vi "点位与索引匹配.vi"(9 "匹配索引号":i32, 10 "配置信息":string[][](table)=[["名称", "点位", "索引号", "逻辑取反"], ["启动按钮", "X100", "0", "0"], ["复位按钮", "X101", "1", "0"], ["暂停按钮", "X102", "2", "0"], ["操作侧安全光栅", "X103", "3", "0"], ["后侧安全光栅", "X104", "4", "0"], ["上层真空检知", "X105", "5", "0"], ["下层真空检知", "X106", "6", "0"], ["上层感应sensor", "X107", "7", "0"], ["下层感应sensor", "X110", "8", "0"], ["传送抓手气缸前位", "X111", "9", "0"], ["传送抓手气缸后位", "X112", "10", "0"], ["上层产品定位气缸前位", "X113", "11", "0"], ["上层产品定位气缸后位", "X114", "12", "0"], ["下层产品定位气缸前位", "X115", "13", "0"], ["下层产品定位气缸后位", "X116", "14", "0"], ["抓手感应产品sensor", "X117", "15", "0"], ["起子1真空检知", "X120", "16", "0"], ["起子2真空检知", "X121", "17", "0"], ["起子3真空检知", "X122", "18", "0"], ["起子4真空检知", "X123", "19", "0"], ["feed01感应sensor", "X124", "20", "0"], ["feed02感应sensor", "X125", "21", "0"], ["feed03感应sensor", "X126", "22", "0"], ["feed04感应sensor", "X127", "23", "0"], ["动子1和2统一坐标sensor", "X130", "24", "0"], ["动子3和4统一坐标sensor", "X131", "25", "0"], ["前后侧统一坐标sensor", "X132", "26", "0"], ["上站允许取料信号", "X133", "27", "0"], ["下站允许投料信号", "X134", "28", "0"], ["上站请求信号", "X135", "29", "0"], ["下站答复信号", "X136", "30", "0"]]) -> (2 "ERROR 2":string)   [LabVIEW 2012]
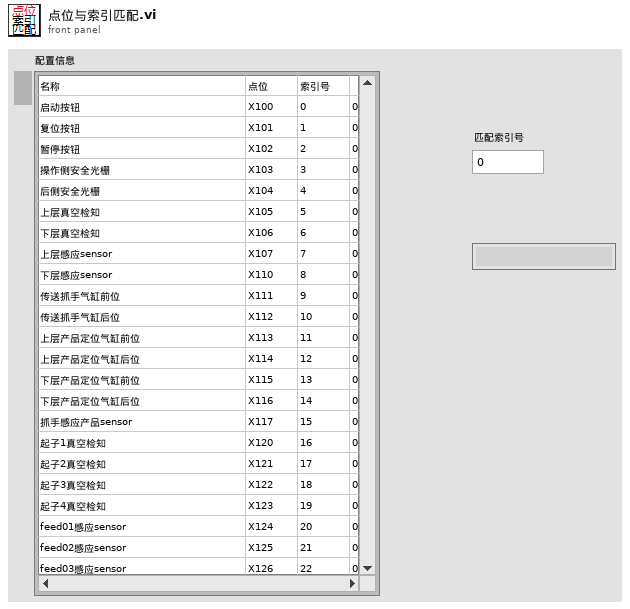
[diagram p1: front panel]
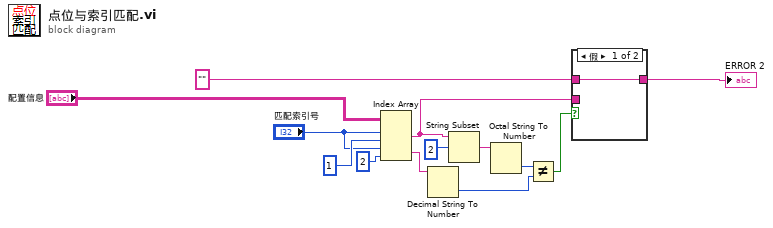
[diagram p0: block diagram]
diagram:
  n1 = Index Array(array="配置信息", index (row) #1="匹配索引号", index (col) #1=1 ("禁用的索引 (列)"), index (row) #2="匹配索引号", index (col) #2=2 ("索引 (列)")) -> (element #1=w1:string, element #2=w4:string)
  n2 = Decimal String To Number(string=w4) -> (number=w7:i32)  [unwired: 2 in, 1 out]
  n3 = String Subset(string=w1, offset (0)=2 ("长度（剩余）")) -> (substring=w9:string)  [unwired: 1 in]
  n4 = Octal String To Number(4:w9) -> (0:w8:u32)  [unwired: 2 in, 1 out]
  n5 = Not Equal?(x=w8, y=w7) -> (x != y?=w3:bool)
  n6 = case shown="假" w3 {
    tunnel: w1 -> [_ w15]
    tunnel: [w14 w15] -> w12
    tunnel: "" -> [w14 _]
    frame False {
    }
    frame True {
    }
  }
  "ERROR 2" <- w12
